vi "Construct_Bad_Track_FOR_(101)_Point-1.vi"(6 "[IN] Indexes for Jumps":i32[](array[numeric]), 7 "[IN] Number of Co\nnnected Points":i32, 8 "error IN":errorcluster, 9 "[IN] Index of recon\nstructed tracks":i32, 10 "[IN] Clusters for Re\nconstructed Tracks":T1, 11 "[IN] Still connected\ntracks in group":T2) -> (0 "error OUT":errorcluster, 2 "[OUT] Clusters for Re\nconstructed Tracks":T1)   [LabVIEW 2013]
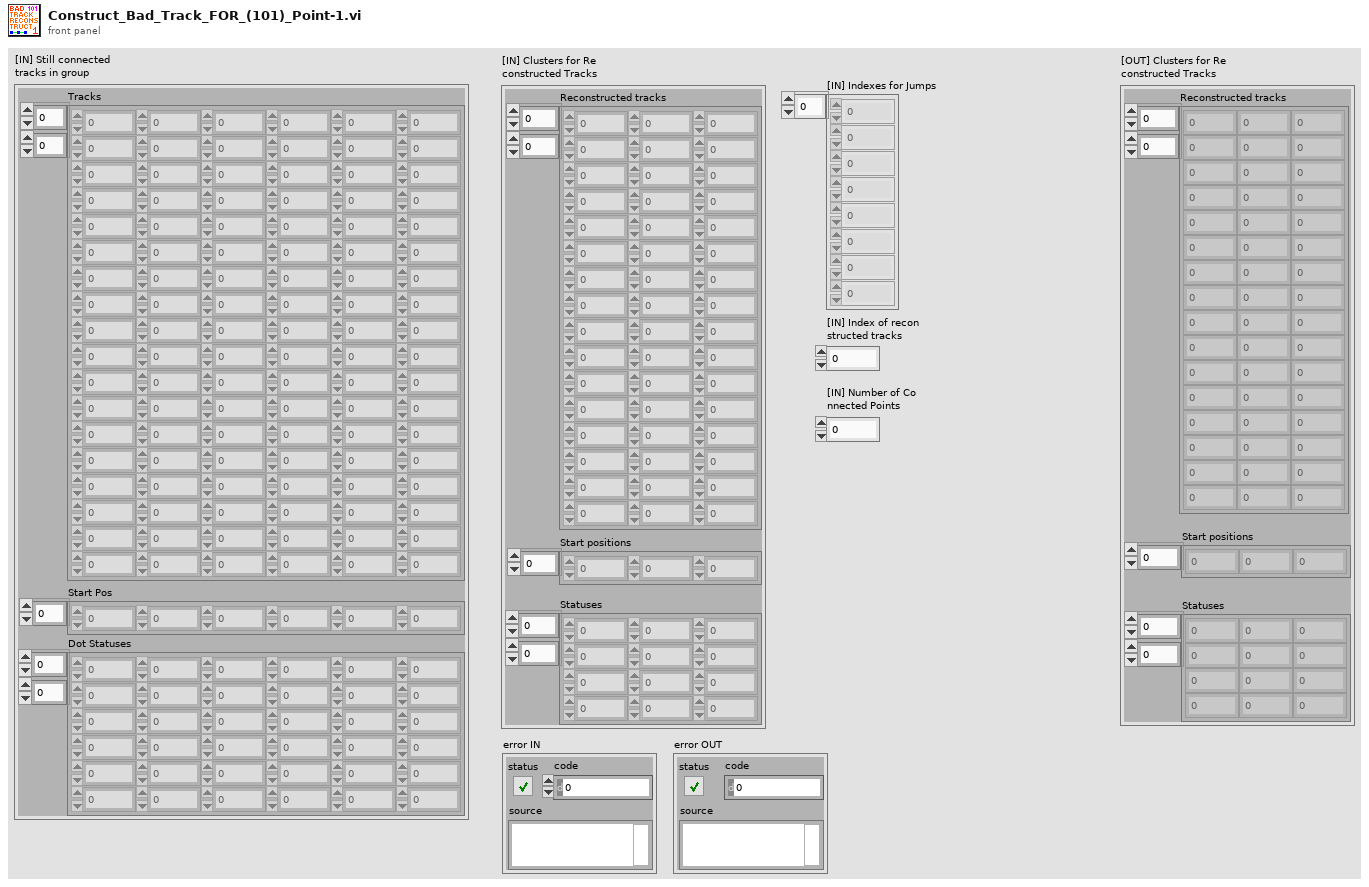
[diagram p1: front panel]
types:
  T1 = cluster{"Reconstructed tracks":dbl[][], "Start positions":i32[], "Statuses":i16[][]}
  T2 = cluster{"Tracks":dbl[][], "Start Pos":i32[], "Dot Statuses":i16[][]}
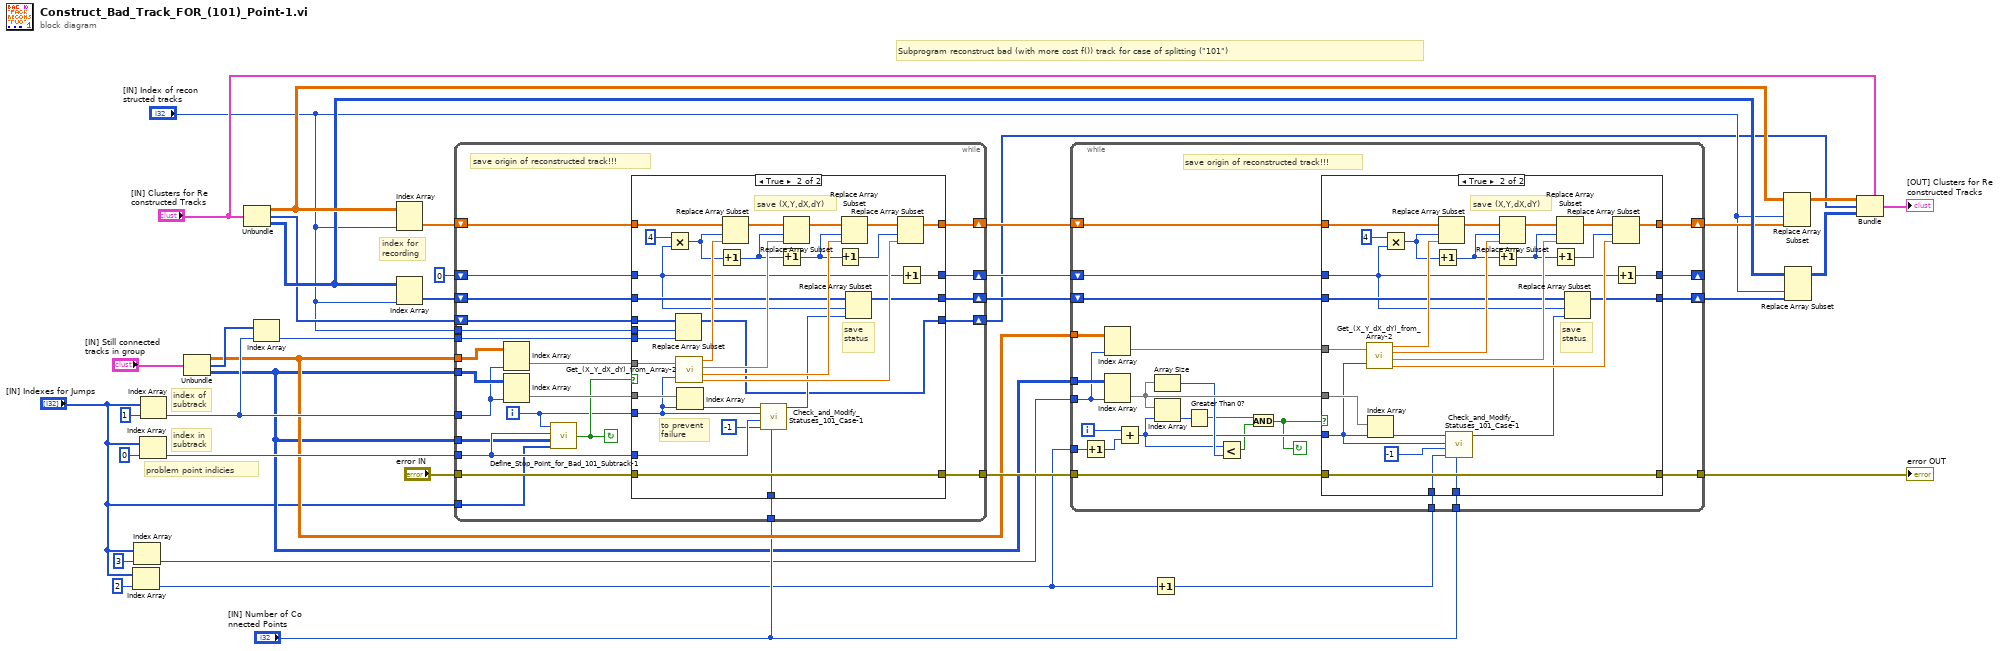
[diagram p0: block diagram]
diagram:
  # "index for\nrecording"
  # "index of\nsubtrack"
  # "index in\nsubtrack"
  # "problem point indicies"
  # "Subprogram reconstruct bad (with more cost f()) track for case of splitting (\"101\")"
  n1 = Index Array(array="[IN] Indexes for Jumps", index=2) -> (element=w6:i32)
  n2 = Index Array(array="[IN] Indexes for Jumps", index=3) -> (element=w9:i32)
  n3 = Index Array(array="[IN] Indexes for Jumps", index=0) -> (element=w26:i32)
  n4 = Index Array(array="[IN] Indexes for Jumps", index=1) -> (element=w29:i32)
  n5 = Unbundle("[IN] Still connected\ntracks in group") -> ("Tracks"=w14:dbl[][], "Start Pos"=w27:i32[], "Dot Statuses"=w8:i16[][])
  n6 = Unbundle("[IN] Clusters for Re\nconstructed Tracks") -> ("Reconstructed tracks"=w33:dbl[][], "Start positions"=w4:i32[], "Statuses"=w32:i16[][])
  n7 = Index Array(array=w27, index=w29) -> (element=w2:i32)
  n8 = Index Array(array=w33, index (col)="[IN] Index of recon\nstructed tracks") -> (element=w25:dbl[])  [unwired: 1 in]
  n9 = Index Array(array=w32, index (col)="[IN] Index of recon\nstructed tracks") -> (element=w24:i16[])  [unwired: 1 in]
  n10 = while {
    tunnel: w26 -> [w43]
    tunnel: w14 -> [w59]
    tunnel: w8 -> [w58]
    tunnel: w29 -> [w57]
    shift-right: [w52] -> w16
    shift-left: w25 -> [w56]
    shift-right: [w50] -> w18
    shift-left: w24 -> [w54]
    shift-right: [w51] -> w17
    shift-left: 0 -> [w53]
    tunnel: "error IN" -> [w49]
    tunnel: [w48] -> w15
    tunnel: "[IN] Number of Co\nnnected Points" -> [w46]
    tunnel: w8 -> [w42]
    tunnel: "[IN] Indexes for Jumps" -> [w41]
    shift-right: [w37] -> w1
    shift-left: w4 -> [w40]
    tunnel: "[IN] Index of recon\nstructed tracks" -> [w39]
    tunnel: w2 -> [w38]
    i -> [w44]
    stop <- w45 continue-if-true
    # "save origin of reconstructed track!!!"
    n11 = Index Array(array=w59, index (col)=w57) -> (element=w55:dbl[])  [unwired: 1 in]
    n12 = Index Array(array=w58, index (col)=w57) -> (element=w47:i16[])  [unwired: 1 in]
    n13 = call "Define_Stop_Point_for_Bad_101_Subtrack-1.vi"("[IN] Indexes for Jumps"=w41, "[IN] Dot Statuses"=w42, "[IN] Index of Mer\nging (\"101\") Point"=w43, "[IN] Current index"=w44) -> ("[OUT] Continue saving points"=w45:bool)
    n14 = case shown="True" w45 {
      tunnel: w56 -> [w64 w93]
      tunnel: w55 -> [_ w95]
      tunnel: w47 -> [_ w94]
      tunnel: w44 -> [_ w73]
      tunnel: w54 -> [w62 w80]
      tunnel: [w62 w79] -> w50
      tunnel: [w64 w78] -> w52
      tunnel: w53 -> [w63 w77]
      tunnel: [w63 w76] -> w51
      tunnel: w49 -> [w61 w75]
      tunnel: [w61 w75] -> w48
      tunnel: w43 -> [_ w72]
      tunnel: w46 -> [_ w71]
      tunnel: w40 -> [w60 w68]
      tunnel: w39 -> [_ w67]
      tunnel: w38 -> [_ w66]
      tunnel: [w60 w65] -> w37
      frame False {
      }
      frame True {
        # "to prevent \nfailure"
        # "save (X,Y,dX,dY)"
        # "save\nstatus"
        n15 = Multiply(x=4, y=w77) -> (x*y=w89:i32)
        n16 = Replace Array Subset(array=w68, new element=w66, index=w67) -> (w65:i32[])
        n17 = call "Get_(X_Y_dX_dY)_from_Array-2.vi"("(X,Y,dX,dY)"=w95, "Index of Displacement"=w73) -> ("X"=w91:dbl, "Y"=w88:dbl, "dX"=w85:dbl, "dY"=w81:dbl)
        n18 = Index Array(array=w94, index=w73) -> (element=w74:i16)
        n19 = Increment(x=w89) -> (x+1=w86:i32)
        n20 = Replace Array Subset(array=w93, new element=w91, index=w89) -> (w90:dbl[])
        n21 = call "Check_and_Modify_Statuses_101_Case-1.vi"("[IN] Number of Co\nnnected Points"=w71, "[IN] Index of Po\nint After \"101\""=-1 ("[IN] Index of Po\nint After \"101\""), "[IN] Index of Pro\nblem \"101\" Point"=w72, "[IN] Current Index"=w73, "[IN] Current Status"=w74) -> ("[OUT] Status"=w70:i16)  [unwired: 4 in]
        n22 = Increment(x=w86) -> (x+1=w84:i32)
        n23 = Replace Array Subset(array=w90, new element=w88, index=w86) -> (w87:dbl[])
        n24 = Increment(x=w84) -> (x+1=w83:i32)
        n25 = Replace Array Subset(array=w87, new element=w85, index=w84) -> (w82:dbl[])
        n26 = Replace Array Subset(array=w80, new element=w70, index=w77) -> (w79:i16[])
        n27 = Replace Array Subset(array=w82, new element=w81, index=w83) -> (w78:dbl[])
        n28 = Increment(x=w77) -> (x+1=w76:i32)
      }
    }
  }
  n29 = Increment(x=w6) -> (x+1=w5:i32)
  n30 = while {
    tunnel: w14 -> [w119]
    tunnel: w8 -> [w118]
    tunnel: w9 -> [w117]
    shift-right: [w112] -> w12
    shift-left: w16 -> [w116]
    shift-right: [w110] -> w11
    shift-left: w18 -> [w114]
    shift-right: [w111] -> _
    shift-left: w17 -> [w113]
    tunnel: w6 -> [w99]
    tunnel: w15 -> [w101]
    tunnel: [w100] -> w10
    tunnel: "[IN] Number of Co\nnnected Points" -> [w97]
    tunnel: w5 -> [w96]
    i -> [w109]
    stop <- w102 continue-if-true
    # "save origin of reconstructed track!!!"
    n31 = Increment(x=w99) -> (x+1=w98:i32)
    n32 = Index Array(array=w119, index (col)=w117) -> (element=w115:dbl[])  [unwired: 1 in]
    n33 = Index Array(array=w118, index (col)=w117) -> (element=w108:i16[])  [unwired: 1 in]
    n34 = Add(x=w109, y=w98) -> (x+y=w105:i32)
    n35 = Array Size(array=w108) -> (size(s)=w106:i32)
    n36 = Index Array(array=w108, index=w105) -> (element=w107:i16)
    n37 = Greater Than 0?(x=w107) -> (x > 0?=w104:bool)
    n38 = Less?(x=w105, y=w106) -> (x < y?=w103:bool)
    n39 = And(x=w104, y=w103) -> (x .and. y?=w102:bool)
    n40 = case shown="True" w102 {
      tunnel: w116 -> [w123 w149]
      tunnel: w115 -> [_ w150]
      tunnel: w108 -> [_ w131]
      tunnel: w105 -> [_ w126]
      tunnel: w114 -> [w121 w136]
      tunnel: [w121 w135] -> w110
      tunnel: [w123 w134] -> w112
      tunnel: w113 -> [w122 w133]
      tunnel: [w122 w132] -> w111
      tunnel: w101 -> [w120 w130]
      tunnel: [w120 w130] -> w100
      tunnel: w97 -> [_ w127]
      tunnel: w96 -> [_ w125]
      frame False {
      }
      frame True {
        # "save (X,Y,dX,dY)"
        # "save\nstatus"
        n41 = call "Get_(X_Y_dX_dY)_from_Array-2.vi"("(X,Y,dX,dY)"=w150, "Index of Displacement"=w126) -> ("X"=w147:dbl, "Y"=w144:dbl, "dX"=w141:dbl, "dY"=w137:dbl)
        n42 = Index Array(array=w131, index=w126) -> (element=w129:i16)
        n43 = Multiply(x=4, y=w133) -> (x*y=w145:i32)
        n44 = Increment(x=w145) -> (x+1=w142:i32)
        n45 = Replace Array Subset(array=w149, new element=w147, index=w145) -> (w146:dbl[])
        n46 = call "Check_and_Modify_Statuses_101_Case-1.vi"("[IN] Number of Co\nnnected Points"=w127, "[IN] Index of Po\nint After \"101\""=w125, "[IN] Index of Pro\nblem \"101\" Point"=-1 ("[IN] Index of Pro\nblem \"101\" Point"), "[IN] Current Index"=w126, "[IN] Current Status"=w129) -> ("[OUT] Status"=w128:i16)  [unwired: 4 in]
        n47 = Increment(x=w142) -> (x+1=w140:i32)
        n48 = Replace Array Subset(array=w146, new element=w144, index=w142) -> (w143:dbl[])
        n49 = Increment(x=w140) -> (x+1=w139:i32)
        n50 = Replace Array Subset(array=w143, new element=w141, index=w140) -> (w138:dbl[])
        n51 = Replace Array Subset(array=w136, new element=w128, index=w133) -> (w135:i16[])
        n52 = Replace Array Subset(array=w138, new element=w137, index=w139) -> (w134:dbl[])
        n53 = Increment(x=w133) -> (x+1=w132:i32)
      }
    }
  }
  "error OUT" <- w10
  n54 = Replace Array Subset(array=w33, new element=w12, index (col)="[IN] Index of recon\nstructed tracks") -> (w21:dbl[][])  [unwired: 1 in]
  n55 = Replace Array Subset(array=w32, new element=w11, index (col)="[IN] Index of recon\nstructed tracks") -> (w22:i16[][])  [unwired: 1 in]
  n56 = Bundle(cluster="[IN] Clusters for Re\nconstructed Tracks", "Reconstructed tracks"=w21, "Start positions"=w1, "Statuses"=w22) -> (→"[OUT] Clusters for Re\nconstructed Tracks":T1)
